vi "Append Delays to Waveform.vi"(8 "error in (no error)":errorcluster, 9 "Post Delay (s)":dbl=0.001 format="%#_6p", 10 "Pre Delay (s)":dbl=0.001 format="%#_6p", 11 "Input Waveform":waveform(dbl)) -> (0 "error out":errorcluster, 3 "Output Waveform":waveform(dbl)(graph))   [LabVIEW 2025, in "TDMS Waveform Creator UI.lvlib"]
uses:
  TDMS Waveform Creator UI.lvlib
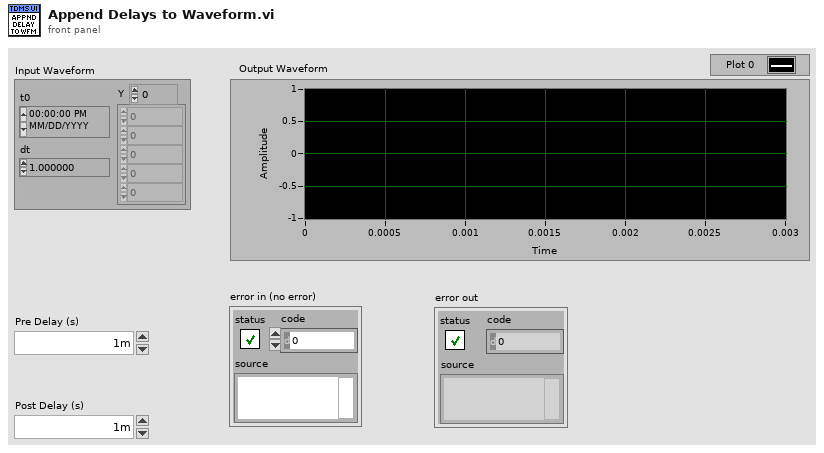
[diagram p1: front panel]
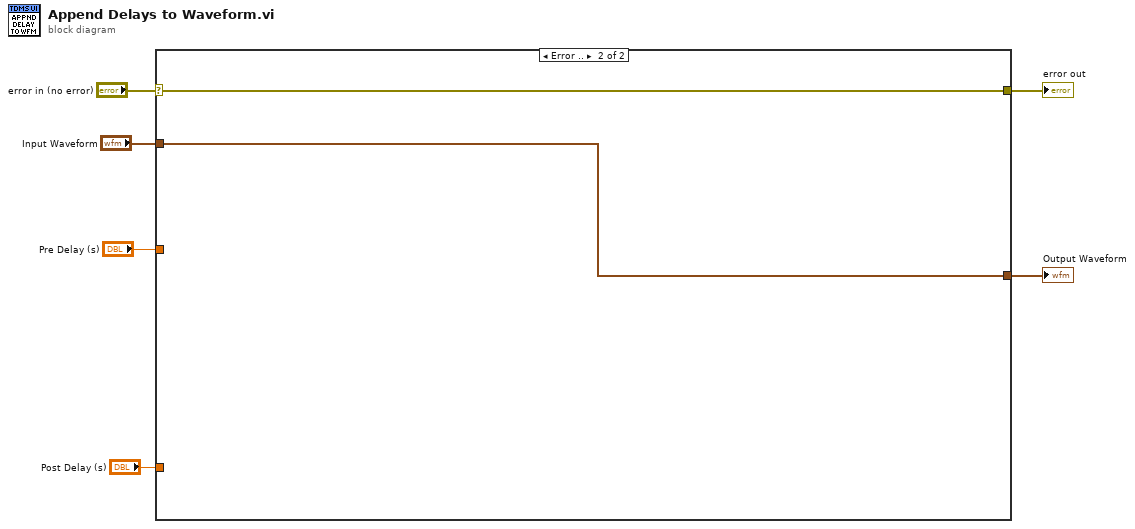
[diagram p0: block diagram]
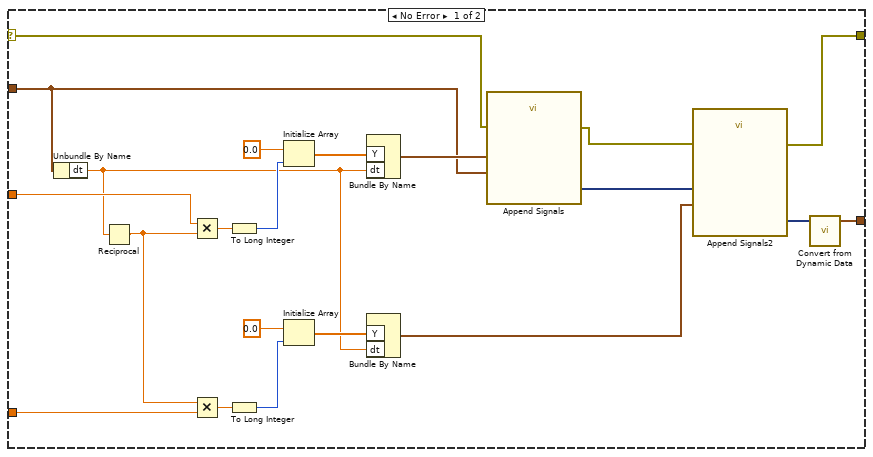
[diagram p2: hidden frame]
diagram:
  n1 = case shown="Error .." "error in (no error)" {
    selector: "error in (no error)" -> [w9 w29]
    tunnel: "Pre Delay (s)" -> [w23 _]
    tunnel: "Post Delay (s)" -> [w20 _]
    tunnel: "Input Waveform" -> [w13 w28]
    tunnel: [w10 w28] -> w3
    tunnel: [w7 w29] -> w1
    frame No Error {
      n2 = Unbundle By Name(w13) -> ("dt"=w11:dbl)
      n3 = Reciprocal(x=w11) -> (1/x=w12:dbl)
      n4 = Multiply(x=w23, y=w12) -> (x*y=w27:dbl)
      n5 = Multiply(x=w12, y=w20) -> (x*y=w19:dbl)
      n6 = To Long Integer(number=w27) -> (32bit integer=w25:i32)
      n7 = To Long Integer(number=w19) -> (32bit integer=w18:i32)
      n8 = Initialize Array(0.0 ("DC Value"), w25) -> (w26:dbl[])
      n9 = Initialize Array(0.0 ("DC Value"), w18) -> (w21:dbl[])
      n10 = Bundle By Name("Y"=w26, "dt"=w11) -> (w17:waveform(dbl))  [unwired: 1 in]
      n11 = Bundle By Name("Y"=w21, "dt"=w11) -> (w15:waveform(dbl))  [unwired: 1 in]
      n12 = call "Append Signals"("error in (no error)"=w9, "Input Signal B"=w13, "Input Signal A"=w17) -> ("error out"=w8:errorcluster, "Appended Signals"=w16:dynamicdata)  [unwired: 7 in]
      n13 = call "Append Signals2"("error in (no error)"=w8, "Input Signal B"=w15, "Input Signal A"=w16) -> ("error out"=w7:errorcluster, "Appended Signals"=w14:dynamicdata)  [unwired: 7 in]
      n14 = call "Convert from Dynamic Data"("Dynamic Data Type"=w14) -> ("Waveform"=w10:waveform(dbl))  [unwired: 3 in]
    }
    frame Error {
    }
  }
  "Output Waveform" <- w3
  "error out" <- w1
